vi "CreateFilePath.vi"(10 "Frame number":i32, 11 "folder":path) -> (3 "Path to file":path)   [LabVIEW 2015]
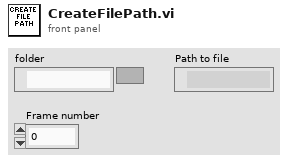
[diagram p1: front panel]
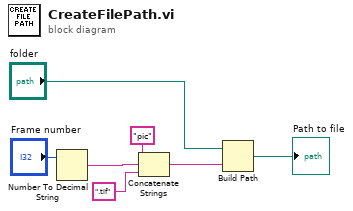
[diagram p0: block diagram]
diagram:
  n1 = Number To Decimal String(number="Frame number") -> (decimal integer string=w2:string)  [unwired: 1 in]
  n2 = Concatenate Strings("pic" ("name or relative path"), w2, ".tif" ("string")) -> (w4:string)
  n3 = Build Path(base path="folder", name or relative path=w4) -> (appended path=→"Path to file":path)
